vi "GetClassListInMemory.vi"(8 "error in (no error)":errorcluster) -> (0 "error out":errorcluster, 3 "Classes in memory":refnum<class>[](array[class]))   [LabVIEW 2020, in "BlueSerialization.lvlib" / "BlueSerializer.lvclass"]
uses:
  BlueSerializer.lvclass
  BlueSerializer.lvclass/BlueSerializer.ctl
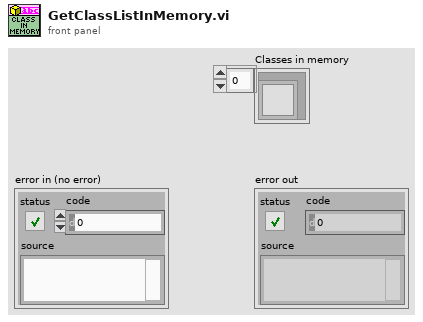
[diagram p1: front panel]
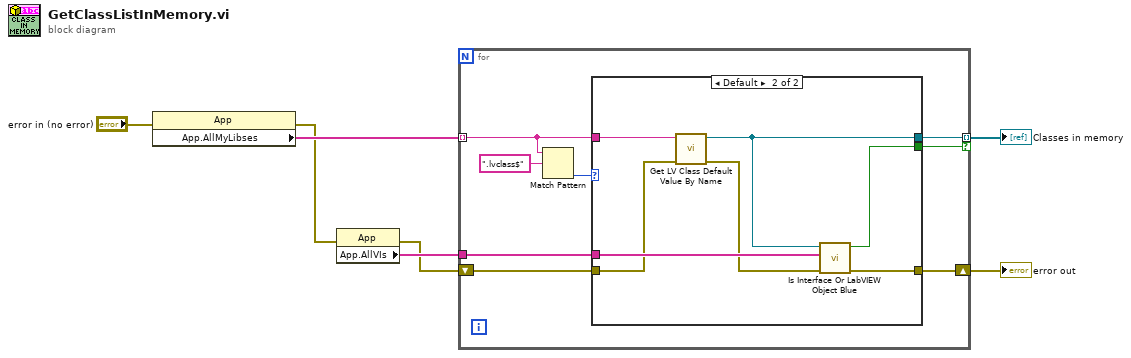
[diagram p0: block diagram]
diagram:
  n1 = property class="App"(error in="error in (no error)") -> (error out=w4:errorcluster, "App.AllMyLibses"=w7:string[])  [unwired: 1 in, 1 out]
  n2 = property class="App"(error in=w4) -> (error out=w3:errorcluster, "App.AllVIs"=w6:string[])  [unwired: 1 in, 1 out]
  n3 = for {
    tunnel: w7 -> [w15] mode=indexing
    tunnel: [w12] -> w2 mode=indexing if=w8
    tunnel: w6 -> [w11]
    shift-right: [w9] -> w1
    shift-left: w3 -> [w10]
    n4 = Match Pattern(string=w15, regular expression=".lvclass$") -> (offset past match=w14:i32)  [unwired: 1 in, 3 out]
    n5 = case shown="Default" w14 {
      tunnel: [_ w21] -> w12
      tunnel: w15 -> [_ w23]
      tunnel: w11 -> [_ w22]
      tunnel: w10 -> [w16 w19]
      tunnel: [w16 w18] -> w9
      tunnel: [_ w17] -> w8
      frame -1 {
      }
      frame Default {
        n6 = call <vilib>:"Get LV Class Default Value By Name.vi"("error in (no error)"=w19, "class name"=w23) -> ("error out"=w20:errorcluster, "object"=w21:refnum<class>)  [unwired: 8 in]
        n7 = call "Is Interface Or LabVIEW Object Blue.vi"("error in (no error)"=w20, "Application:All VIs In Memory"=w22, "LabVIEW Object"=w21) -> ("error out"=w18:errorcluster, "Is Class?"=w17:bool)  [unwired: 7 in]
      }
    }
  }
  "Classes in memory" <- w2
  "error out" <- w1
